vi "Remove Line.vi"(8 "error in":errorcluster, 10 "Active Line Name":string, 11 "Objects":T1) -> (0 "error out":errorcluster)   [LabVIEW 2014, in "tag bus configurable plugin editor node.lvclass"]
uses:
  tag bus configurable plugin editor node.lvclass
  Table Manager/object ref.ctl
  Configuration Editor/Classes/Engine Parent/Engine Parent Editor Node.lvclass
  Configuration Editor/Classes/Module editor node/module editor node.lvclass
  module/configuration/tag bus configurable plugin module configuration.lvclass
  <vilib>/NI/Configuration Framework/serializable configuration/NISE_CEF_serializable configuration.lvclass/NISE_CEF_serializable configuration.ctl
  <vilib>/Utility/LVClass/Get LV Class Name.vi
  <vilib>/NI/Configuration Framework/error generator/NISE_error generator.vi
  <vilib>/NI/Configuration Framework/serializable configuration/NISE_CEF_serializable configuration.lvclass
  Table Manager/Table Manager.lvclass
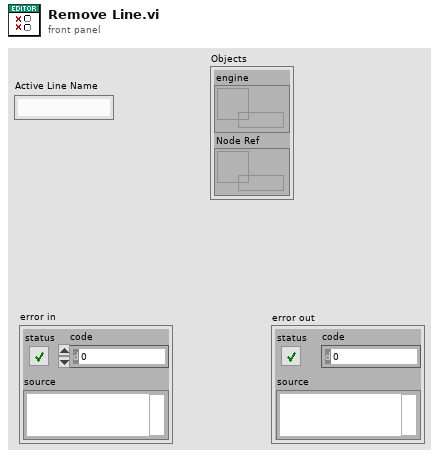
[diagram p1: front panel]
types:
  T1 = typedef "Table Manager.lvlib/Table Manager.lvclass/object ref.ctl" = cluster{"engine":refnum<data-value>, "Node Ref":refnum<data-value>}
  T2 = typedef "tag bus configurable plugin module configuration.lvclass/Line.ctl" = cluster{"channel":refnum<class "TBM channel.lvclass">}
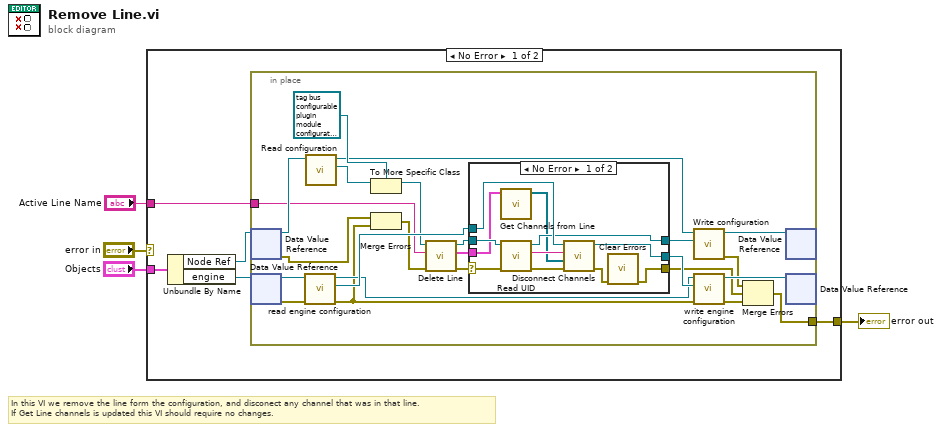
[diagram p0: block diagram]
diagram:
  # "In this VI we remove the line form the configuration, and disconect any channel that was in that line.\nIf Get Line channels is updated this VI should require no changes."
  n1 = case shown="No Error" "error in" {
    selector: "error in" -> [_ w48]
    tunnel: "Objects" -> [w8 _]
    tunnel: [w9 w48] -> w3
    tunnel: "Active Line Name" -> [w5 _]
    frame No Error {
      n2 = Unbundle By Name(w8) -> ("Node Ref"=w6:refnum<data-value>, "engine"=w7:refnum<data-value>)
      n3 = in-place {
        in-place-border: [w12] -> w9
        in-place-border: w5 -> [w19]
        n4 = in-place-dvr #1(w6) -> (w25:refnum<class "module editor node.lvclass">, w26:errorcluster)
        n5 = in-place-dvr #2(w7) -> (w31:refnum<class "Engine Parent Editor Node.lvclass">, w30:errorcluster)
        n6 = call "read engine configuration.vi"("error in"=w30, "Engine Parent Editor Node in"=w31) -> ("error out"=w27:errorcluster, "engine configuration"=w29:refnum<class "engine configuration.lvclass">, "Engine Parent Editor Node out"=w28:refnum<class "Engine Parent Editor Node.lvclass">)  [unwired: 7 in]
        n7 = call-dynamic "Read configuration.vi"("NISE_CEF_serializable node in"=w25) -> ("configuration"=w23:refnum<class "NISE_CEF_serializable configuration.lvclass">, "NISE_CEF_serializable node out"=w21:refnum<class "module editor node.lvclass">)  [unwired: 8 in, 1 out]
        n8 = To More Specific Class(target class=refnum<class "tag bus configurable plugin module configuration.lvclass"> refnum ("tag bus configurable plugin module configuration out"), reference=w23) -> (specific class reference=w18:refnum<class "tag bus configurable plugin module configuration.lvclass">)  [unwired: 1 in, 1 out]
        n9 = Merge Errors(w26, w27) -> (w16:errorcluster)
        n10 = call "Delete Line.vi"("error in"=w16, "Active Line Name"=w19, "tag bus configurable plugin module configuration in"=w18) -> ("error out"=w15:errorcluster, "deleted line"=w10:T2, "tag bus configurable plugin module configuration out"=w17:refnum<class "tag bus configurable plugin module configuration.lvclass">)  [unwired: 6 in]
        n11 = case shown="No Error" w15 {
          selector: w15 -> [w38 w45]
          tunnel: w17 -> [w42 w46]
          tunnel: w29 -> [w44 w47]
          tunnel: [w43 w47] -> w32
          tunnel: [w39 w46] -> w20
          tunnel: [w34 w45] -> w11
          tunnel: w10 -> [w37 _]
          frame No Error {
            n12 = call "Get Channels from Line.vi"("Line"=w37) -> ("Array"=w36:refnum<class "TBM channel.lvclass">[])  [unwired: 10 in]
            n13 = call <vilib>:"Read UID.vi"("error in"=w38, "configuration in"=w42) -> ("error out"=w40:errorcluster, "instance id"=w41:string, "configuration out"=w39:refnum<class "tag bus configurable plugin module configuration.lvclass">)  [unwired: 7 in]
            n14 = call "Disconnect Channels.vi"("error in (no error)"=w40, "Deleted Channels"=w36, "instance id"=w41, "engine configuration in"=w44) -> ("error out"=w35:errorcluster, "engine configuration out"=w43:refnum<class "engine configuration.lvclass">)  [unwired: 6 in]
            n15 = call <vilib>:"Clear Errors.vi"("error in (no error)"=w35) -> ("error out"=w34:errorcluster)  [unwired: 5 in, 1 out]
          }
          frame Error {
          }
        }
        n16 = call-dynamic "Write configuration.vi"("configuration"=w20, "NISE_CEF_serializable node in"=w21) -> ("error out"=w14:errorcluster, "NISE_CEF_serializable node out"=w22:refnum<class "module editor node.lvclass">)  [unwired: 8 in]
        n17 = call "write engine configuration.vi"("error in"=w27, "engine configuration"=w32, "Engine Parent Editor Node in"=w28) -> ("error out"=w13:errorcluster, "Engine Parent Editor Node out"=w33:refnum<class "Engine Parent Editor Node.lvclass">)  [unwired: 7 in]
        n18 = Merge Errors(w14, w11, w13) -> (w12:errorcluster)
        n19 = in-place-dvr #1(w22) -> ()  [unwired: 2 out]
        n20 = in-place-dvr #2(w33) -> ()  [unwired: 2 out]
      }
    }
    frame Error {
    }
  }
  "error out" <- w3
